vi "Eat.vi"(8 "error in (no error)":errorcluster, 11 "Animal In":refnum<class "Animal.lvclass">) -> (0 "error out":errorcluster, 2 "Result":string, 3 "Animal Out":refnum<class "Animal.lvclass">)   [LabVIEW 2020, in "Animal.lvclass"]
doc: "All animals can eat and in general an animal is not hungry after eating."
uses:
  Animal.lvclass
  Animal.lvclass/Animal.ctl
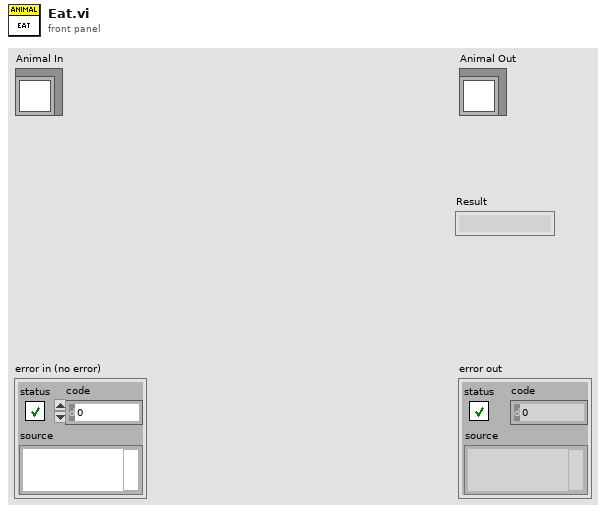
[diagram p1: front panel]
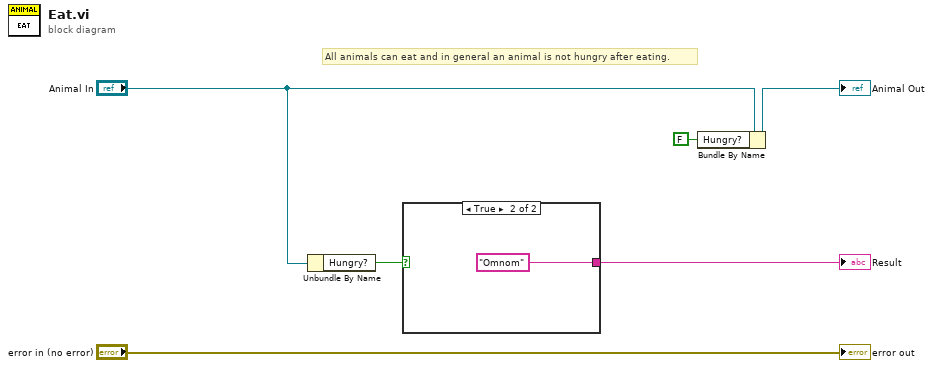
[diagram p0: block diagram]
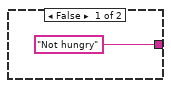
[diagram p2: hidden frame]
diagram:
  # "All animals can eat and in general an animal is not hungry after eating."
  n1 = Unbundle By Name("Animal In") -> ("Hungry?"=w3:bool)
  n2 = case shown="True" w3 {
    tunnel: ["Not hungry" ("Result") "Omnom" ("Result")] -> w2
    frame False {
    }
    frame True {
    }
  }
  "Result" <- w2
  n3 = Bundle By Name(cluster="Animal In", "Hungry?"=FALSE) -> (→"Animal Out":refnum<class "Animal.lvclass">)
  "error out" <- "error in (no error)"
